vi "查询clonm对应的所有内容.vi"(7 "条件":enum16{"DISTINCT", "MIN", "MAX"}(ring), 8 "error in (no error)":errorcluster caption="错误输入（无错误）", 9 "组合框":string(combo), 10 "database":string="database1.mdb", 11 "table":string(combo)="CODMn") -> (0 "error out":errorcluster caption="错误输出", 3 "输出数组":string[](array[string]))   [LabVIEW 2016]
uses:
  <vilib>/Utility/sysdir.llb/System Directory Type.ctl
  <vilib>/addons/database/Connection.llb/DB Tools Open Connec (String).vi
  <vilib>/addons/database/Connection.llb/Conn Execute.vi
  <vilib>/addons/database/Recordset.llb/Rec Fetch Recordset Data (R).vi
  <vilib>/addons/database/Recordset.llb/Rec Destroy - Connection.vi
  <vilib>/addons/database/_DB Variant To Data/Database Variant To Data.xnode
  <vilib>/addons/database/NI_Database_API.lvlib
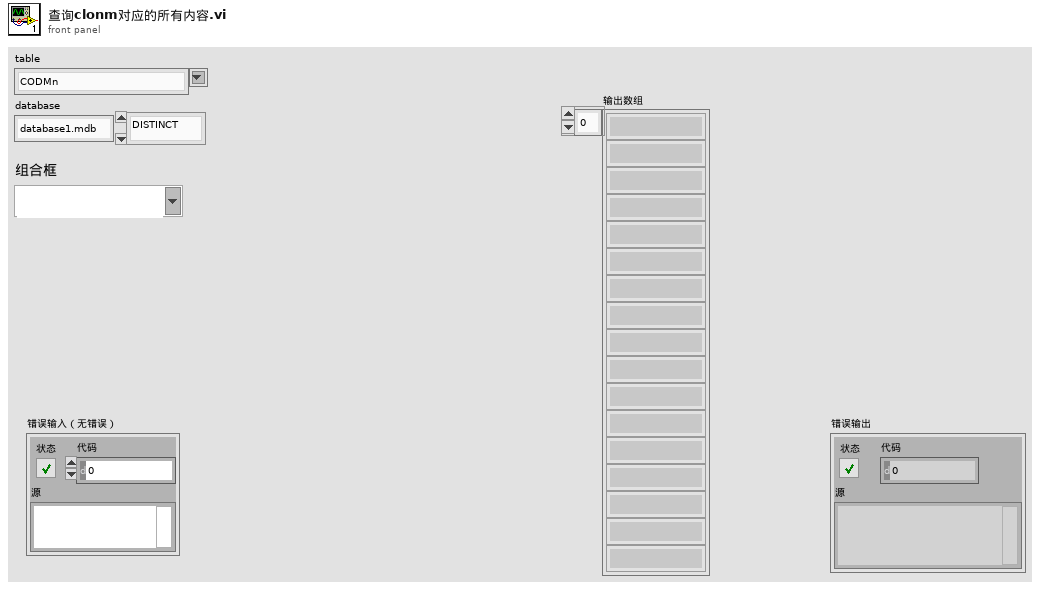
[diagram p1: front panel]
types:
  T1 = typedef "System Directory Type.ctl" = i32
  T2 = typedef "NI_Database_API.lvlib/Conn ObjectReference.ctl" = refnum<k1>
  T3 = typedef "NI_Database_API.lvlib/Rec ObjectReference.ctl" = refnum<k1>
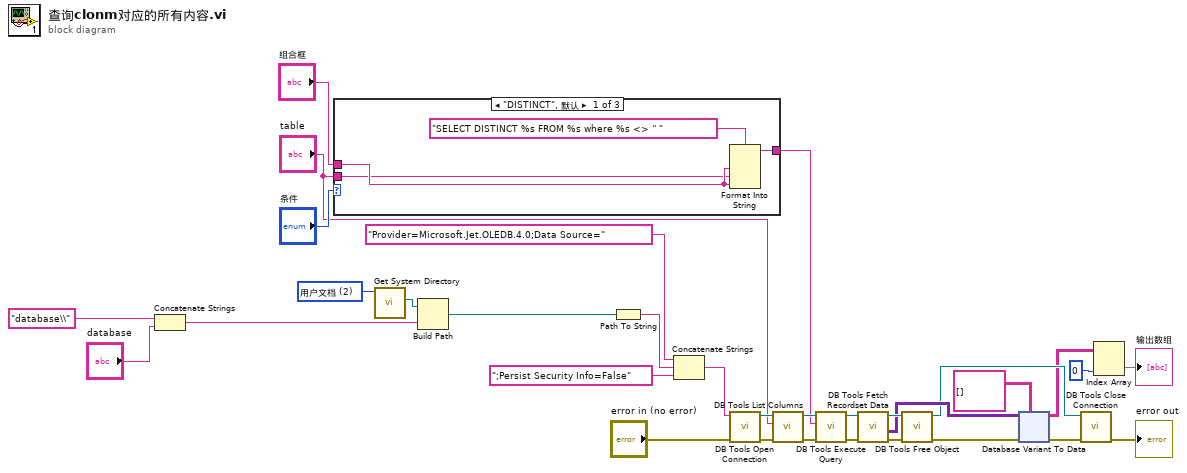
[diagram p0: block diagram]
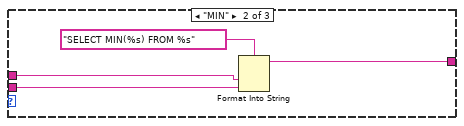
[diagram p2: hidden frame]
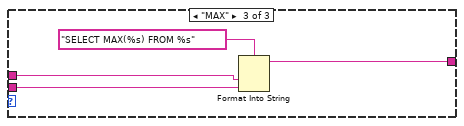
[diagram p3: hidden frame]
diagram:
  w1 = T1 2 items=["用户目录"=0, "用户桌面"=1, "用户文档"=2, "用户应用程序数据"=3, "用户设置"=4, "用户临时目录"=5, "公共文档"=6, "公共应用程序数据"=7, "公共设置"=8, "公共缓存"=13, "系统核心库"=9, "系统安装库"=10, "应用程序文件"=11, "启动盘根目录"=12] ("system directory type")
  n1 = Concatenate Strings("database\\" ("名称或相对路径"), "database") -> (w25:string)
  n2 = case shown="\"DISTINCT\", 默认" "条件" {
    tunnel: [w36 w37 w41] -> w4
    tunnel: "组合框" -> [w34 w38 w43]
    tunnel: "table" -> [w33 w39 w42]
    frame "DISTINCT", Default {
      n3 = Format Into String(format string="SELECT DISTINCT %s FROM %s where %s <> '' ", w34, w33, w34) -> (resulting string=w36:string)  [unwired: 2 in, 1 out]
    }
    frame "MIN" {
      n4 = Format Into String(format string="SELECT MIN(%s) FROM %s", w38, w39) -> (resulting string=w37:string)  [unwired: 2 in, 1 out]
    }
    frame "MAX" {
      n5 = Format Into String(format string="SELECT MAX(%s) FROM %s", w43, w42) -> (resulting string=w41:string)  [unwired: 2 in, 1 out]
    }
  }
  n6 = call <vilib>:"Get System Directory.vi"("system directory type"=w1) -> ("system directory"=w2:path)  [unwired: 10 in]
  n7 = Build Path(base path=w2, name or relative path=w25) -> (appended path=w24:path)
  n8 = Path To String(path=w24) -> (string=w28:string)
  n9 = Concatenate Strings("Provider=Microsoft.Jet.OLEDB.4.0;Data Source=", w28, ";Persist Security Info=False") -> (w22:string)
  n10 = call-poly <vilib>:"DB Tools Open Connection.vi"("error in (no error)"="error in (no error)", "connection information"=w22) -> ("error out"=w31:errorcluster, "connection reference"=w32:T2)  [unwired: 6 in]
  n11 = call <vilib>:"DB Tools List Columns.vi"("error in (no error)"=w31, "table"="table", "connection reference"=w32) -> ("error out"=w10:errorcluster, "connection reference out"=w11:T2)  [unwired: 1 in, 2 out]
  n12 = call-poly <vilib>:"DB Tools Execute Query.vi"("error in (no error)"=w10, "SQL query"=w4, "connection reference"=w11) -> ("error out"=w20:errorcluster, "recordset reference"=w21:T3)  [unwired: 5 in]
  n13 = call-poly <vilib>:"DB Tools Fetch Recordset Data.vi"("error in (no error)"=w20, "recordset reference"=w21) -> ("error out"=w19:errorcluster, "recordset data"=w15:variant[][], "recordset reference out"=w18:T3)  [unwired: 3 in]
  n14 = call-poly <vilib>:"DB Tools Free Object.vi"("error in (no error)"=w19, "recordset reference"=w18) -> ("error out"=w14:errorcluster, "connection reference"=w13:T2)  [unwired: 8 in]
  n15 = xnode "Database Variant To Data"("database variant"=w15, "error in (no error)"=w14, "type"=string[][] []) -> ("data"=w9:string[][], "error out"=w16:errorcluster)
  n16 = call <vilib>:"DB Tools Close Connection.vi"("error in (no error)"=w16, "connection reference"=w13) -> ("error out"=→"error out":errorcluster)  [unwired: 5 in]
  n17 = Index Array(array=w9, index (col)=0 ("禁用的索引 (列)")) -> (element=→"输出数组":string[])  [unwired: 1 in]
